vi "Scan Barcode.vi"(11 "Bypass Validation":bool) -> (0 "Next DUT?":bool, 1 "Valid?":bool, 2 "Reason":string, 3 "Barcode out":string)   [LabVIEW 2021, in "Sequence Engine.lvlib"]
uses:
  Sequence Engine.lvlib
panel:
  out "Barcode 2":string
  in  "Close":bool
  out "Serial Number":string
  out "Year Code":string
  out "Week Code":string
  out "Customer Model":string
  out "Deltron Code":string
  in  "Barcode":string
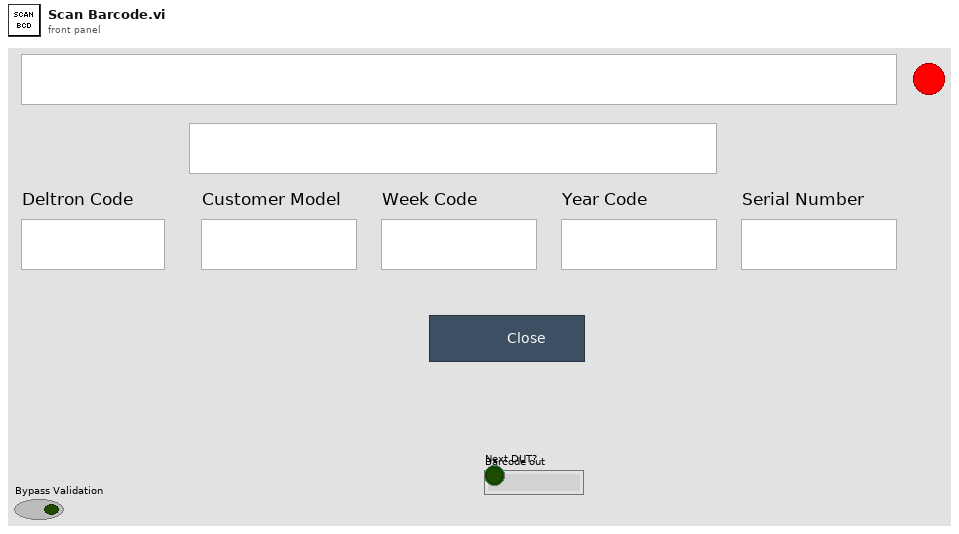
[diagram p1: front panel]
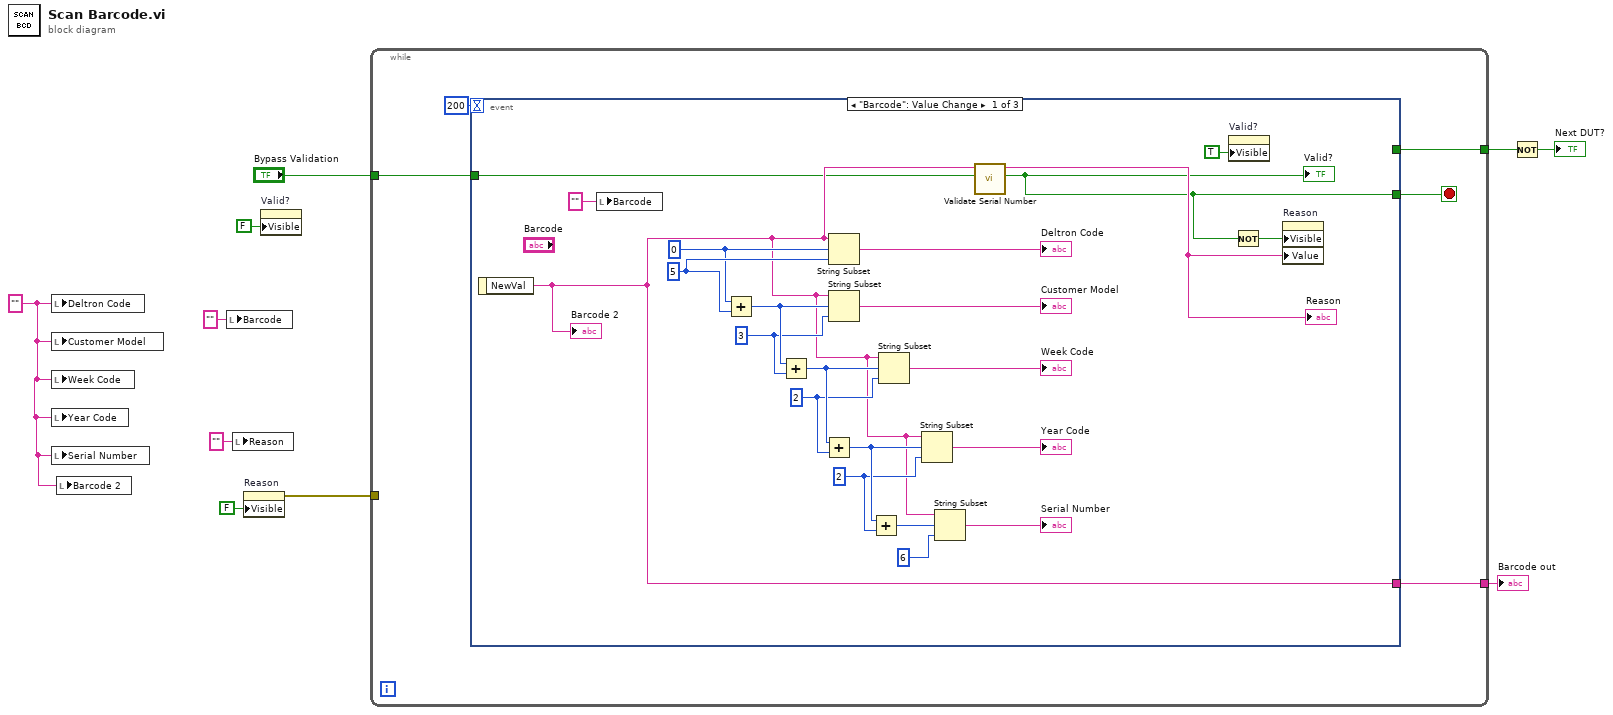
[diagram p0: block diagram]
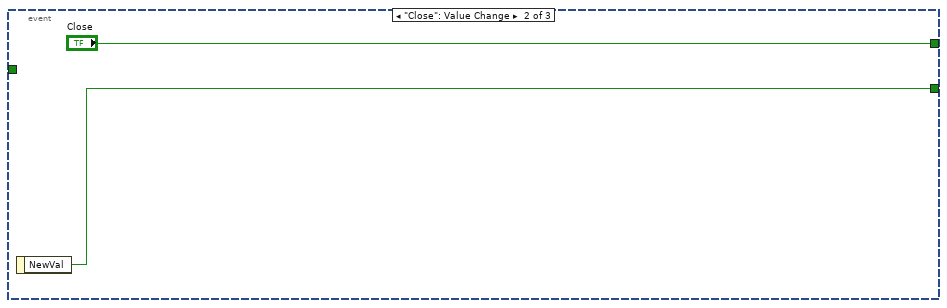
[diagram p2: hidden frame]
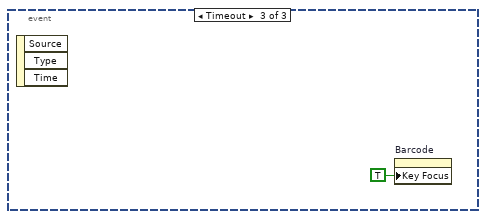
[diagram p3: hidden frame]
diagram:
  w2 = "" ("Deltron Code")
  n1 = local write "Deltron Code"(w2) -> ()
  n2 = local write "Customer Model"(w2) -> ()
  n3 = local write "Week Code"(w2) -> ()
  n4 = local write "Year Code"(w2) -> ()
  n5 = local write "Serial Number"(w2) -> ()
  n6 = local write "Barcode 2"(w2) -> ()
  n7 = local write "Barcode"("" ("Barcode")) -> ()
  n8 = local write "Reason"("" ("Reason")) -> ()
  n9 = property on="Reason" class="Str"("Visible"=FALSE) -> (error out=w7:errorcluster)  [unwired: 2 in, 1 out]
  n10 = property on="Valid?" class="Bool (strict)"("Visible"=FALSE) -> ()  [unwired: 2 in, 2 out]
  n11 = while {
    tunnel: w7 -> [_]
    tunnel: [w13] -> w6
    tunnel: [w12] -> w5
    tunnel: "Bypass Validation" -> [w11]
    stop <- w15 stop-if-true
    n12 = event shown="[0] \"Barcode\": Value Change" {
      selector: _ -> [_ _ _]
      dyn-events: _ -> [_ _ _]
      timeout: 200 -> [_ _ _]
      tunnel: [w20 w39 _] -> w15
      tunnel: [w17 _ _] -> w13
      tunnel: [_ "Close" _] -> w12
      tunnel: w11 -> [w16 _ _]
      event "Barcode": Value Change {
        w28 = 2 ("length (rest)")
        w26 = 2 ("length (rest)")
        w25 = 3 ("length (rest)")
        w24 = 5 ("length (rest)")
        w23 = 0 ("offset (0)")
        n13 = event-data() -> ("NewVal"=w17:string)  [unwired: 1 in]
        "Barcode 2" <- w17
        n14 = local write "Barcode"("" ("Barcode")) -> ()
        n15 = Add(x=w23, y=w24) -> (x+y=w31:i32)
        n16 = Add(x=w31, y=w25) -> (x+y=w33:i32)
        n17 = Add(x=w33, y=w26) -> (x+y=w36:i32)
        n18 = String Subset(string=w17, offset (0)=w23, length (rest)=w24) -> (substring=→"Deltron Code":string)
        n19 = String Subset(string=w17, offset (0)=w31, length (rest)=w25) -> (substring=→"Customer Model":string)
        n20 = Add(x=w36, y=w28) -> (x+y=w37:i32)
        n21 = String Subset(string=w17, offset (0)=w33, length (rest)=w26) -> (substring=→"Week Code":string)
        n22 = String Subset(string=w17, offset (0)=w36, length (rest)=w28) -> (substring=→"Year Code":string)
        n23 = String Subset(string=w17, offset (0)=w37, length (rest)=6 ("length (rest)")) -> (substring=→"Serial Number":string)
        n24 = call "Validate Serial Number.vi"("Bypass Validation"=w16, "Serial Number"=w17) -> ("Valid SrNo?"=w20:bool, "Reason"=w21:string)  [unwired: 8 in]
        "Reason" <- w21
        "Valid?" <- w20
        n25 = property on="Valid?" class="Bool (strict)"("Visible"=TRUE) -> ()  [unwired: 2 in, 2 out]
        n26 = Not(x=w20) -> (.not. x?=w22:bool)
        n27 = property on="Reason" class="Str"("Visible"=w22, "Value"=w21) -> ()  [unwired: 2 in, 2 out]
      }
      event "Close": Value Change {
        n28 = event-data() -> ("NewVal"=w39:bool)  [unwired: 1 in]
      }
      event Timeout {
        n29 = event-data() -> ()  [unwired: 1 in, 3 out]
        n30 = property on="Barcode" class="Str"("Key Focus"=TRUE) -> ()  [unwired: 2 in, 2 out]
      }
    }
  }
  "Barcode out" <- w6
  n31 = Not(x=w5) -> (.not. x?=→"Next DUT?":bool)
